vi "Setup Statically-Linked subWorkers.vi"(8 "error in":errorcluster, 11 "Camera detection in":refnum<class "Camera detection.lvclass">) -> (0 "error out":errorcluster, 3 "Camera detection out":refnum<class "Camera detection.lvclass">)   [LabVIEW 2026, in "Camera detection.lvclass"]
doc: "This VI performs a setup of all the statically-linked subWorkers that belong to the Worker that owns this VI. This VI must be called <b>before</b> any statically-linked subWorkers are called."
uses:
  Camera detection.lvclass
  Camera detection.lvclass/Camera detection.ctl
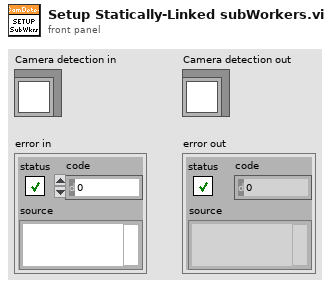
[diagram p1: front panel]
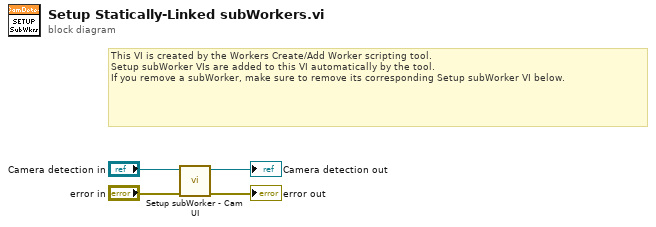
[diagram p0: block diagram]
diagram:
  # "This VI is created by the Workers Create/Add Worker scripting tool.\nSetup subWorker VIs are added to this VI automatically by the tool.\nIf you remove a subWorker, make sure to remove its corresponding Setup subWorker VI below."
  n1 = call "Setup subWorker - Cam UI.vi"("error in"="error in", "Camera detection in"="Camera detection in") -> ("error out"=→"error out":errorcluster, "Camera detection out"=→"Camera detection out":refnum<class "Camera detection.lvclass">)  [unwired: 8 in]
